vi "Handle Messages.vi"(8 "error in (no error)":errorcluster, 9 "Message Data":variant, 10 "Message":string, 11 "Cashier In":refnum<class "Cashier.lvclass">) -> (0 "error out":errorcluster, 3 "Cashier Out":refnum<class "Cashier.lvclass">)   [LabVIEW 2020, in "Cashier.lvclass"]
uses:
  Cashier.lvclass
  C:/git/astemes-triarc-examples/source/Coffee Shop/Processes/People/Person/Person.lvclass
  Support/Order/Order.lvclass
  Person/Person.lvclass/Person.ctl
  Worker/Worker.lvclass
  Customers/Customer/Customer.lvclass
  Person/Person.lvclass
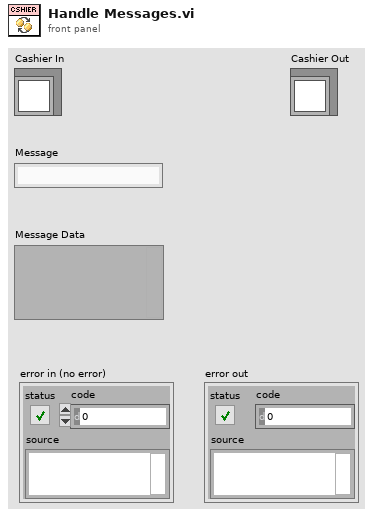
[diagram p1: front panel]
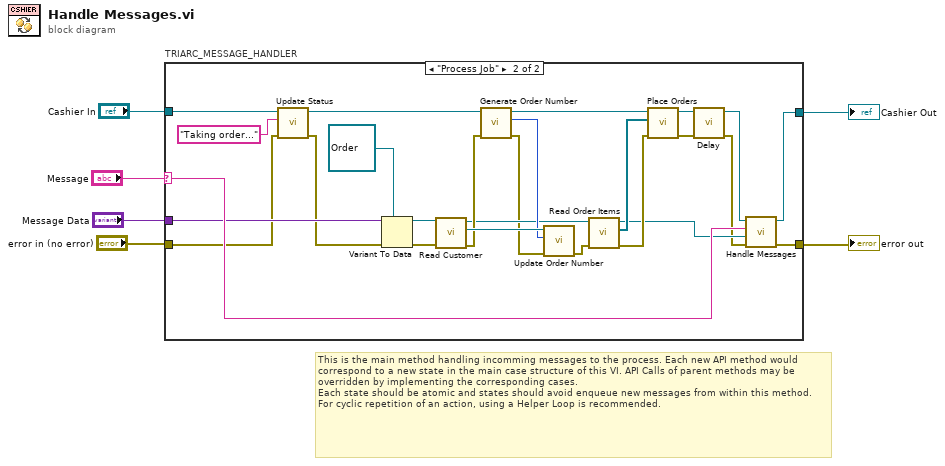
[diagram p0: block diagram]
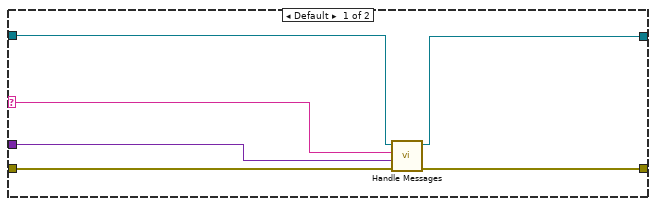
[diagram p2: hidden frame]
diagram:
  # "This is the main method handling incomming messages to the process. Each new API method would correspond to a new state in the main case structure of this VI. API Calls of parent methods may be overridden by implementing the corresponding cases.\nEach state should be atomic and states should avoid enqueue new messages from within this method. For cyclic repetition of an action, using a Helper Loop is recommended."
  n1 = case "TRIARC_MESSAGE_HANDLER" shown="\"Process Job\"" "Message" {
    selector: "Message" -> [w10 w37]
    tunnel: "error in (no error)" -> [w9 w30]
    tunnel: "Cashier In" -> [w12 w38]
    tunnel: "Message Data" -> [w11 w34]
    tunnel: [w8 w36] -> w2
    tunnel: [w7 w35] -> w1
    frame Default {
      n2 = call-parent "Handle Messages.vi"("error in (no error)"=w9, "Message Data"=w11, "Message"=w10, "Worker In"=w12) -> ("error out"=w8:errorcluster, "Worker Out"=w7:refnum<class "Cashier.lvclass">)  [unwired: 6 in]
    }
    frame "Process Job" {
      n3 = call "Update Status.vi"("error in (no error)"=w30, "Status"="Taking order..." ("Message"), "Person In"=w38) -> ("error out"=w31:errorcluster, "Person Out"=w32:refnum<class "Cashier.lvclass">)  [unwired: 7 in]
      n4 = Variant To Data(error in=w31, type=refnum<class "Order.lvclass"> refnum ("Order.lvclass"), Variant=w34) -> (data=w29:refnum<class "Order.lvclass">, error out=w26:errorcluster)
      n5 = call-dynamic "Read Customer.vi"("error in (no error)"=w26, "Order in"=w29) -> ("error out"=w25:errorcluster, "Customer"=w28:refnum<class "Customer.lvclass">, "Order out"=w24:refnum<class "Order.lvclass">)  [unwired: 7 in]
      n6 = call "Generate Order Number.vi"("error in (no error)"=w25, "Cashier in"=w32) -> ("error out"=w23:errorcluster, "Order Number"=w27:u32, "Cashier out"=w21:refnum<class "Cashier.lvclass">)  [unwired: 7 in]
      n7 = call "Update Order Number.vi"("error in (no error)"=w23, "Order Number"=w27, "Customer In"=w28) -> ("error out"=w22:errorcluster)  [unwired: 7 in, 1 out]
      n8 = call-dynamic "Read Order Items.vi"("error in (no error)"=w22, "Order in"=w24) -> ("error out"=w19:errorcluster, "Items"=w20:refnum<class "Order Item.lvclass">[], "Order out"=w18:refnum<class "Order.lvclass">)  [unwired: 7 in]
      n9 = call "Place Orders.vi"("error in (no error)"=w19, "Items"=w20, "Cashier in"=w21) -> ("error out"=w14:errorcluster, "Cashier out"=w16:refnum<class "Cashier.lvclass">)  [unwired: 7 in]
      n10 = call "Delay.vi"("error in (no error)"=w14, "Person In"=w16) -> ("error out"=w13:errorcluster, "Person Out"=w15:refnum<class "Cashier.lvclass">)  [unwired: 8 in]
      n11 = call-parent "Handle Messages.vi"("error in (no error)"=w13, "Message Data"=w18, "Message"=w37, "Worker In"=w15) -> ("error out"=w36:errorcluster, "Worker Out"=w35:refnum<class "Cashier.lvclass">)  [unwired: 6 in]
    }
  }
  "error out" <- w2
  "Cashier Out" <- w1
